vi "1038 Timer.vi"(9 "Reset?":bool, 11 "Time Target":dbl=2.5 format="%#_13g") -> (3 "Done?":bool)   [LabVIEW 2015]
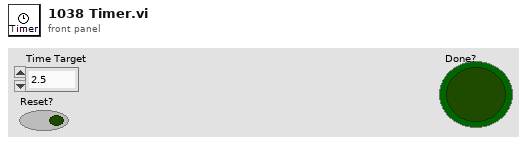
[diagram p1: front panel]
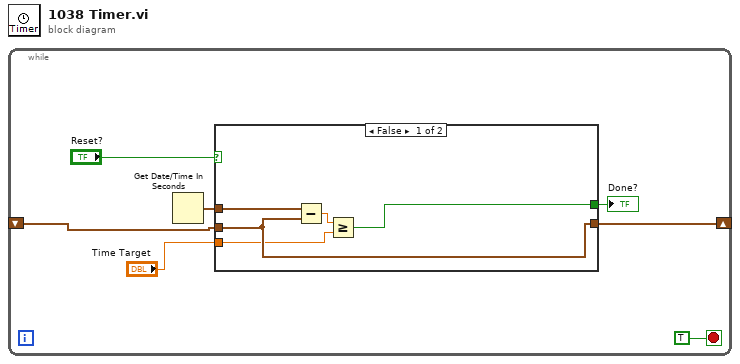
[diagram p0: block diagram]
diagram:
  n1 = while {
    shift-right: [w6] -> _
    shift-left: _ -> [w4]
    stop <- TRUE stop-if-true
    n2 = Get Date/Time In Seconds() -> (seconds since 1Jan1904=w7:timestamp)
    n3 = case shown="False" "Reset?" {
      tunnel: w7 -> [w12 w13]
      tunnel: [w9 w13] -> w6
      tunnel: w4 -> [w9 _]
      tunnel: [w10 _] -> w2
      tunnel: "Time Target" -> [w8 _]
      frame False {
        n4 = Subtract(x=w12, y=w9) -> (x-y=w11:dbl)
        n5 = Greater Or Equal?(x=w11, y=w8) -> (x >= y?=w10:bool)
      }
      frame True {
      }
    }
    "Done?" <- w2
  }
